vi "Popup Date-Time.vi"(8 "error in (no error)":errorcluster, 9 "Panel":refnum<class "Panel.lvclass">, 10 "String in":string, 11 "Numeric Data Type in":refnum<class "Numeric Data Type.lvclass">) -> (0 "error out":errorcluster, 2 "String out":string, 3 "Numeric Data Type out":refnum<class "Numeric Data Type.lvclass">)   [LabVIEW 2018, in "Numeric Data Type.lvclass"]
uses:
  Numeric Data Type.lvclass
  <vilib>/MGI/Panel Manager/Panel/Panel/Panel.lvclass
  Numeric Data Type.lvclass/Numeric Data Type.ctl
  <vilib>/Utility/miscctls.llb/LVPointTypeDef.ctl
panel:
  in  "Time Stamp":timestamp format="%<%Y/%m/%d>T"
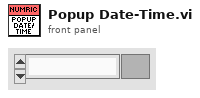
[diagram p1: front panel]
types:
  T1 = typedef "Numeric Data Type.lvclass/Response to Values Outside of Limits Enum.ctl" = enum16{"Ignore", "Coerce to nearest", "Coerce up", "Coerce down"}
  T2 = typedef "LVPointTypeDef.ctl" = cluster{"Horizontal":i16, "Vertical":i16}
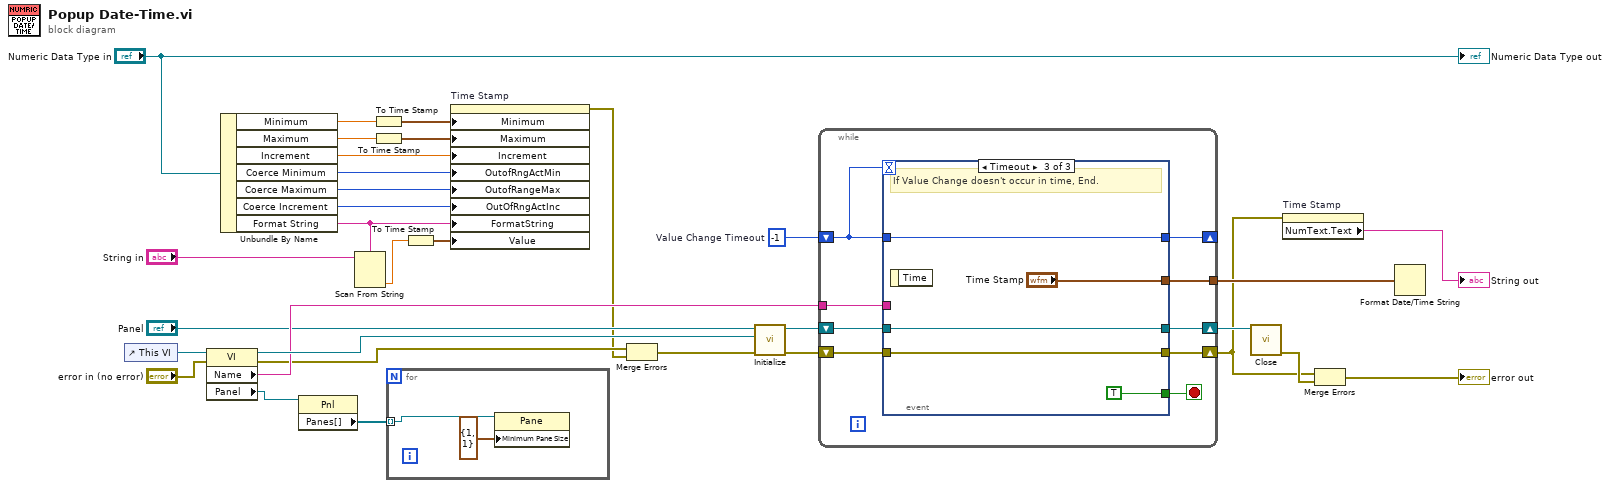
[diagram p0: block diagram]
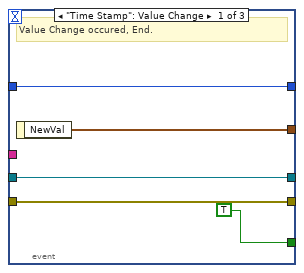
[diagram p2: hidden frame]
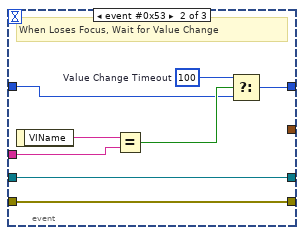
[diagram p3: hidden frame]
diagram:
  w32 = -1  # Value Change Timeout
  n1 = control-ref of="This VI"() -> (w29:refnum<vi>)
  n2 = property class="VI"(reference=w29, error in="error in (no error)") -> (reference out=w28:refnum<vi>, error out=w21:errorcluster, "Name"=w27:string, "Panel"=w11:refnum<vi>)
  n3 = Unbundle By Name("Numeric Data Type in") -> ("Minimum"=w20:dbl, "Maximum"=w19:dbl, "Increment"=w18:dbl, "Coerce Minimum"=w17:T1, "Coerce Maximum"=w16:T1, "Coerce Increment"=w15:T1, "Format String"=w7:string)
  n4 = property class="Pnl"(reference=w11) -> ("Panes[]"=w10:refnum<vi>[])  [unwired: 1 in, 2 out]
  n5 = Scan From String(format string=w7, input string="String in") -> (output 1=w5:dbl)  [unwired: 3 in, 3 out]
  n6 = To Time Stamp(1:w20) -> (0:w9:timestamp)
  n7 = To Time Stamp(1:w19) -> (0:w8:timestamp)
  n8 = for {
    tunnel: w10 -> [w34] mode=indexing
    n9 = property class="Pane"(reference=w34, "Minimum Pane Size"=T2 {"Horizontal"=1, "Vertical"=1}) -> ()  [unwired: 1 in, 2 out]
  }
  n10 = To Time Stamp(1:w5) -> (0:w4:timestamp)
  n11 = property on="Time Stamp" class="AbsTime (strict)"("Minimum"=w9, "Maximum"=w8, "Increment"=w18, "OutofRngActMin"=w17, "OutofRangeMax"=w16, "OutOfRngActInc"=w15, "FormatString"=w7, "Value"=w4) -> (error out=w13:errorcluster)  [unwired: 2 in, 1 out]
  n12 = Merge Errors(w21, w13) -> (w14:errorcluster)
  n13 = call <vilib>:"Initialize.vi"("error in (no error)"=w14, "VI Refnum"=w28, "Panel In"="Panel") -> ("error out"=w30:errorcluster, "Panel Out"=w31:refnum<class "Panel.lvclass">)  [unwired: 6 in, 1 out]
  n14 = while {
    shift-right: [w43] -> w1
    shift-left: w30 -> [w42]
    shift-right: [w40] -> w25
    shift-left: w31 -> [w39]
    tunnel: [w38] -> w3
    tunnel: w27 -> [w37]
    shift-right: [w35] -> _
    shift-left: w32 -> [w36]
    stop <- w41 stop-if-true
    n15 = event shown="[2] Timeout" {
      selector: _ -> [_ _ _]
      dyn-events: _ -> [_ _ _]
      timeout: w36 -> [_ _ _]
      tunnel: [w45 w54 w59] -> w43
      tunnel: w42 -> [w45 w54 w59]
      tunnel: [TRUE _ TRUE] -> w41
      tunnel: [w47 w53 w60] -> w40
      tunnel: w39 -> [w47 w53 w60]
      tunnel: [w46 _ "Time Stamp"] -> w38
      tunnel: w37 -> [_ w55 _]
      tunnel: w36 -> [w44 w50 w57]
      tunnel: [w44 w49 w57] -> w35
      event "Time Stamp": Value Change {
        # "Value Change occured, End."
        n16 = event-data() -> ("NewVal"=w46:timestamp)  [unwired: 1 in]
      }
      event event #0x53 {
        w51 = 100  # Value Change Timeout
        # "When Loses Focus, Wait for Value Change"
        n17 = event-data() -> ("VIName"=w56:string)  [unwired: 1 in]
        n18 = Equal?(x=w56, y=w55) -> (x = y?=w52:bool)
        n19 = Select(t=w51, s=w52, f=w50) -> (s? t:f=w49:i32)
      }
      event Timeout {
        # "If Value Change doesn't occur in time, End."
        n20 = event-data() -> ()  [unwired: 1 in, 1 out]
      }
    }
  }
  n21 = call-dynamic "Close.vi"("Panel In"=w25) -> ("Error Out"=w26:errorcluster)  [unwired: 10 in]
  n22 = property on="Time Stamp" class="AbsTime (strict)"(error in=w1) -> ("NumText.Text"=→"String out":string)  [unwired: 1 in, 2 out]
  n23 = Merge Errors(w1, w26) -> (→"error out":errorcluster)
  n24 = Format Date/Time String(seconds (now)=w3) -> ()  [unwired: 2 in, 1 out]
  "Numeric Data Type out" <- "Numeric Data Type in"
